vi "LANnumber.vi"(8 "error in (no error)":errorcluster, 11 "search udp":string="irisudp") -> (0 "error out":errorcluster, 3 "LAN number":i32)   [LabVIEW 2018]
panel:
  out "array":string[](array[string])
  out "standard output":string
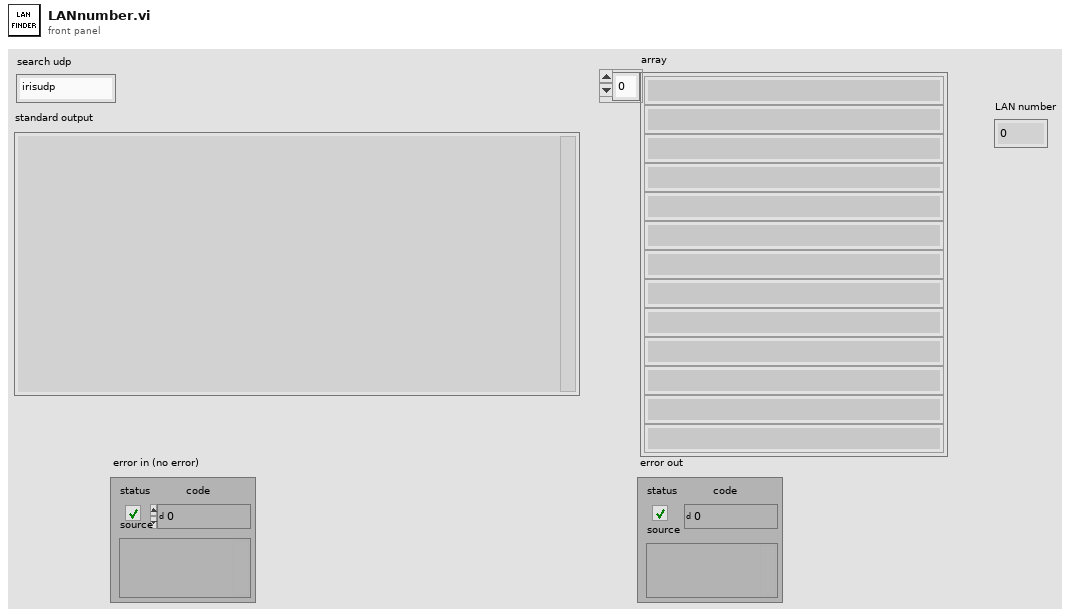
[diagram p1: front panel]
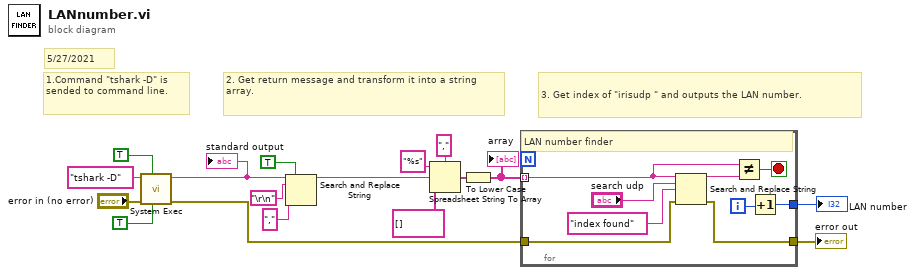
[diagram p0: block diagram]
diagram:
  # "5/27/2021"
  # "3. Get index of \"irisudp \" and outputs the LAN number."
  # "2. Get return message and transform it into a string array."
  # "1.Command \"tshark -D\" is sended to command line."
  n1 = call "System Exec.vi"("run minimized? (F)"=TRUE, "wait until completion? (T)"=TRUE, "error in (no error)"="error in (no error)", "command line"="tshark -D") -> ("error out"=w5:errorcluster, "standard output"=w11:string)  [unwired: 4 in, 2 out]
  "standard output" <- w11
  n2 = Search and Replace String(replace all?=TRUE ("replace all? (F)"), input string=w11, search string="\r\n", replace string="," ("replace string (\"\")")) -> (result string=w9:string)  [unwired: 4 in, 3 out]
  n3 = Spreadsheet String To Array(delimiter (Tab)=",", format string="%s", spreadsheet string=w9, array type (2D Dbl)=string[] []) -> (array=w2:string[])
  n4 = To Lower Case(string=w2) -> (all lower case string=w1:string[])
  "array" <- w1
  n5 = for {
    tunnel: w1 -> [w24] mode=indexing
    tunnel: [w22] -> w6
    tunnel: w5 -> [w19]
    tunnel: [w18] -> w4
    i -> [w26]
    stop <- w20 stop-if-true
    # "LAN number finder"
    n6 = Search and Replace String(input string=w24, search string="search udp", replace string="index found" ("replace string (\"\")"), error in=w19) -> (result string=w21:string, error out=w18:errorcluster)  [unwired: 4 in, 2 out]
    n7 = Not Equal?(x=w24, y=w21) -> (x != y?=w20:bool)
    n8 = Increment(x=w26) -> (x+1=w22:i32)
  }
  "error out" <- w4
  "LAN number" <- w6
